vi "Check Lockin Settings.vi"(7 "Number of channels":i32, 8 "error in (no error)":errorcluster, 11 "Lock-in settings":T1={"Sine Frequency, Hz"=0.0, "Time constant, s"=0.12500000000000006, "Low-pass filter"=enum."No filtering", "Output representation"=enum."Real/Imaginary", "Phases, deg"=[], "Low-pass filter Order"=1, "Decimating factor"=1, "Samples to Read"=10000, "Post-filter decimation"=1, "Blocks to average"=1, "Trig delay, points"=0, "Harmonics per channel"=[], "Amplitude scale"=enum."RMS"} {"Time constant, s" format="%.1e"}) -> (0 "error out":errorcluster, 3 "Lock-in settings out":T1={"Sine Frequency, Hz"=0.0, "Time constant, s"=0.12500000000000006, "Low-pass filter"=enum."No filtering", "Output representation"=enum."Real/Imaginary", "Phases, deg"=[], "Low-pass filter Order"=1, "Decimating factor"=1, "Samples to Read"=10000, "Post-filter decimation"=1, "Blocks to average"=1, "Trig delay, points"=0, "Harmonics per channel"=[], "Amplitude scale"=enum."RMS"} {"Time constant, s" format="%.1e"})   [LabVIEW 2015]
uses:
  Controls/Lockin Settings.ctl
  Controls/Harmonics per channel.ctl
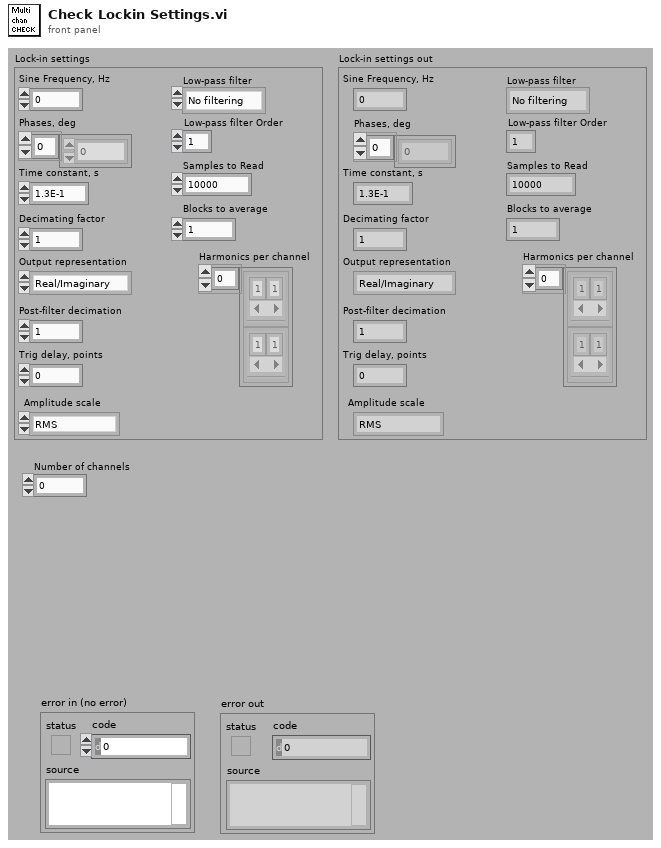
[diagram p1: front panel]
types:
  T1 = typedef "Lockin Settings.ctl" = cluster{"Sine Frequency, Hz":dbl, "Time constant, s":dbl, "Low-pass filter":enum16{"No filtering", "Butterworth", "Bessel"}, "Output representation":enum16{"Real/Imaginary", "Polar"}, "Phases, deg":dbl[], "Low-pass filter Order":i32, "Decimating factor":i32, "Samples to Read":i32, "Post-filter decimation":i32, "Blocks to average":i32, "Trig delay, points":i32, "Harmonics per channel":T2, "Amplitude scale":enum16{"Amplitude", "RMS", "Peak-to-Peak"}}
  T2 = typedef "Harmonics per channel.ctl" = cluster{"Harmonics":i32[]}[]
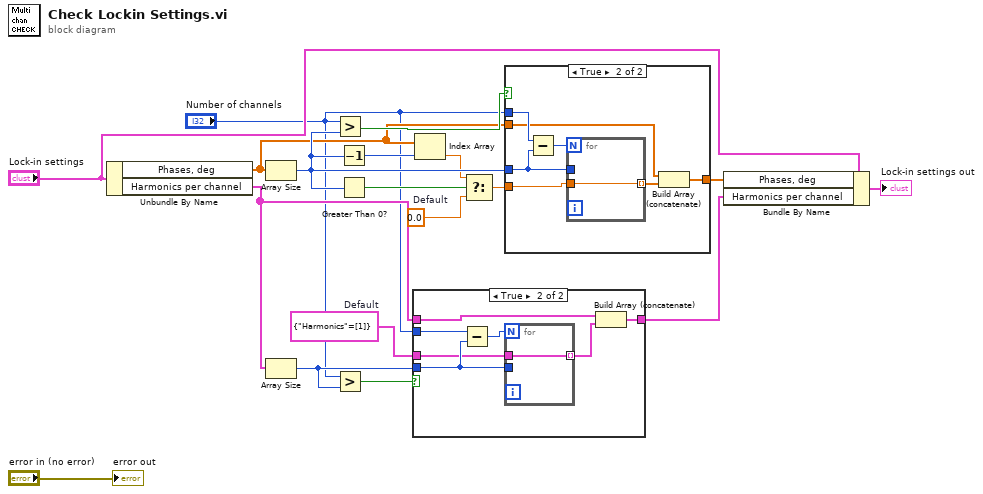
[diagram p0: block diagram]
diagram:
  w3 = cluster{"Harmonics":i32[]} {"Harmonics"=[1]}  # Default
  w11 = 0.0  # Default
  n1 = Unbundle By Name("Lock-in settings") -> ("Phases, deg"=w12:dbl[], "Harmonics per channel"=w5:T2)
  n2 = Array Size(array=w12) -> (size(s)=w16:i32)
  n3 = Array Size(array=w5) -> (size(s)=w6:i32)
  n4 = Greater?(x="Number of channels", y=w16) -> (0:w18:bool)
  n5 = Greater?(x="Number of channels", y=w6) -> (0:w7:bool)
  n6 = Decrement(x=w16) -> (x-1=w17:i32)
  n7 = Greater Than 0?(x=w16) -> (x > 0?=w15:bool)
  n8 = case shown="True" w7 {
    tunnel: "Number of channels" -> [_ w26]
    tunnel: w6 -> [_ w23]
    tunnel: w5 -> [w19 w24]
    tunnel: [w19 w21] -> w2
    tunnel: w3 -> [_ w20]
    frame False {
    }
    frame True {
      n9 = Subtract(x=w26, y=w23) -> (x-y=w22:i32)
      n10 = for {
        N: w22 -> [_]
        tunnel: [w27] -> w25 mode=indexing
        tunnel: w23 -> [_]
        tunnel: w20 -> [w27]
      }
      n11 = Build Array (concatenate)(w24, w25) -> (w21:T2)
    }
  }
  n12 = Index Array(array=w12, index=w17) -> (element=w14:dbl)
  n13 = Select(t=w14, s=w15, f=w11) -> (s? t:f=w13:dbl)
  n14 = case shown="True" w18 {
    tunnel: "Number of channels" -> [_ w35]
    tunnel: w16 -> [_ w32]
    tunnel: w12 -> [w28 w33]
    tunnel: [w28 w30] -> w8
    tunnel: w13 -> [_ w29]
    frame False {
    }
    frame True {
      n15 = Subtract(x=w35, y=w32) -> (x-y=w31:i32)
      n16 = for {
        N: w31 -> [_]
        tunnel: [w36] -> w34 mode=indexing
        tunnel: w32 -> [_]
        tunnel: w29 -> [w36]
      }
      n17 = Build Array (concatenate)(w33, w34) -> (w30:dbl[])
    }
  }
  n18 = Bundle By Name(cluster="Lock-in settings", "Phases, deg"=w8, "Harmonics per channel"=w2) -> (→"Lock-in settings out":T1)
  "error out" <- "error in (no error)"
